vi "fibonacci.vi"() -> ()   [LabVIEW 2014]
panel:
  out "Array":dbl[](array[numeric])
  in  "Numeric":dbl
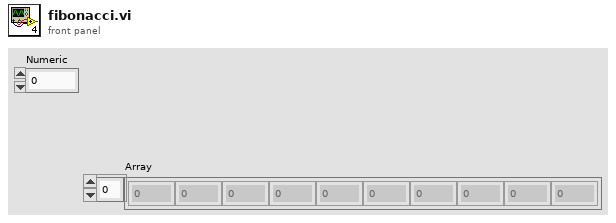
[diagram p1: front panel]
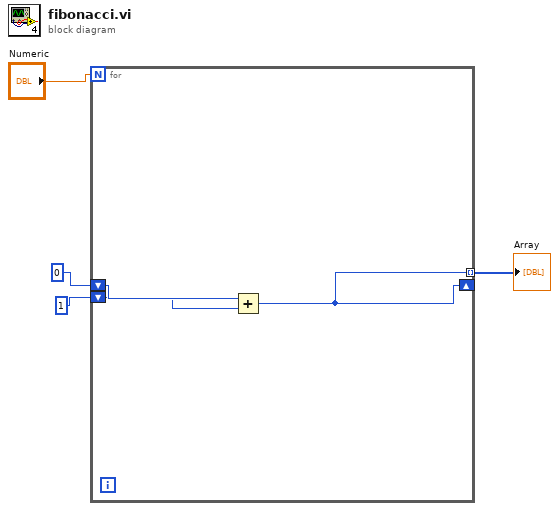
[diagram p0: block diagram]
diagram:
  n1 = for {
    N: "Numeric" -> [_]
    shift-right: [w5] -> _
    shift-left: 0 -> [w7]
    shift-left: 1 -> [w6]
    tunnel: [w5] -> w1 mode=indexing
    n2 = Add(x=w7, y=w6) -> (x+y=w5:i32)
  }
  "Array" <- w1
